vi "CreateAllQueues.vi"(8 "error in (no error)":errorcluster) -> (0 "error IO":errorcluster, 3 "output cluster":T1)   [LabVIEW 2014]
uses:
  Controls/Queues.ctl
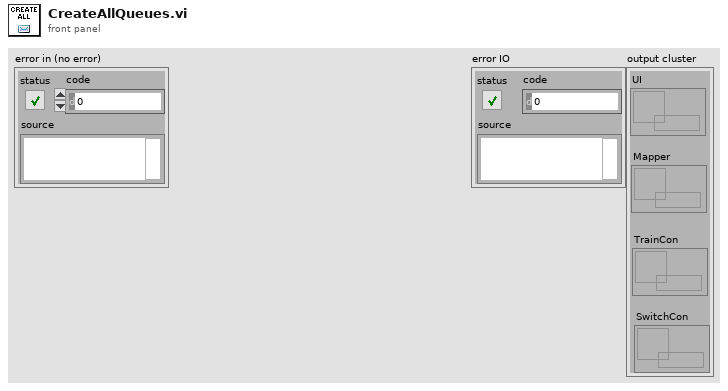
[diagram p1: front panel]
types:
  T1 = typedef "Queues.ctl" = cluster{"UI":refnum<queue>, "Mapper":refnum<queue>, "TrainCon":refnum<queue>, "SwitchCon":refnum<queue>}
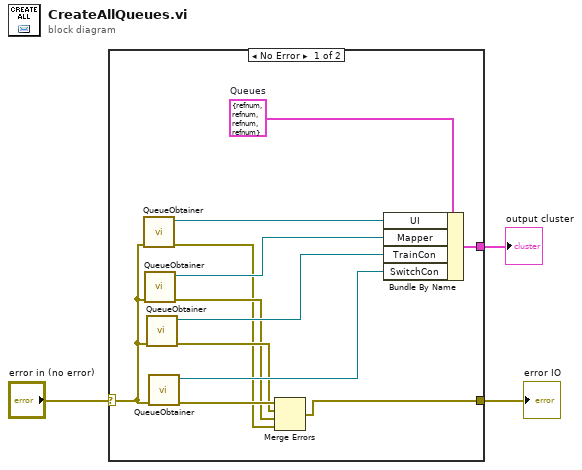
[diagram p0: block diagram]
diagram:
  n1 = case shown="No Error" "error in (no error)" {
    selector: "error in (no error)" -> [w6 w16]
    tunnel: [w5 w16] -> w2
    tunnel: [w4 _] -> w1
    frame No Error {
      w15 = T1 {"UI"=refnum, "Mapper"=refnum, "TrainCon"=refnum, "SwitchCon"=refnum}  # Queues
      n2 = call "QueueObtainer.vi"("error in (no error)"=w6) -> ("error out"=w7:errorcluster, "queue out"=w14:refnum<queue>)  [unwired: 9 in]
      n3 = call "QueueObtainer.vi"("error in (no error)"=w6) -> ("error out"=w8:errorcluster, "queue out"=w11:refnum<queue>)  [unwired: 9 in]
      n4 = call "QueueObtainer.vi"("error in (no error)"=w6) -> ("error out"=w9:errorcluster, "queue out"=w12:refnum<queue>)  [unwired: 9 in]
      n5 = call "QueueObtainer.vi"("error in (no error)"=w6) -> ("error out"=w10:errorcluster, "queue out"=w13:refnum<queue>)  [unwired: 9 in]
      n6 = Merge Errors(w10, w9, w8, w7) -> (w5:errorcluster)
      n7 = Bundle By Name(cluster=w15, "UI"=w14, "Mapper"=w11, "TrainCon"=w12, "SwitchCon"=w13) -> (w4:T1)
    }
    frame Error {
    }
  }
  "error IO" <- w2
  "output cluster" <- w1
